vi "Create Control Addon.vi"(8 "error in (no error)":errorcluster, 11 "Name":string) -> (0 "error out":errorcluster, 3 "Custom Device Ref":refnum<k24>)   [LabVIEW 2013, in "Control SysDef API.lvlib"]
uses:
  Control SysDef API.lvlib
  NationalInstruments.VeriStand.SystemDefinitionAPI
  Shared/Constants.vi
  Shared/Control Addon Shared.lvlib
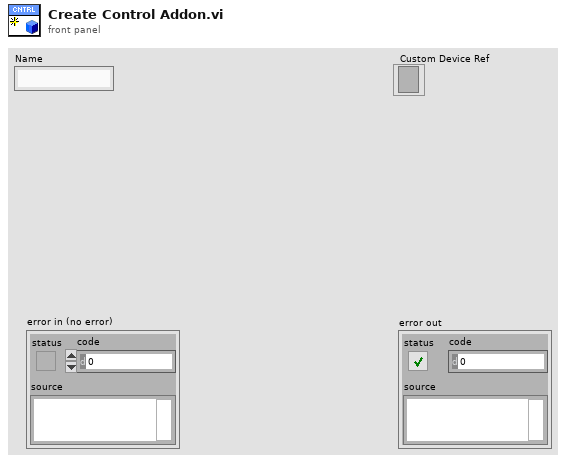
[diagram p1: front panel]
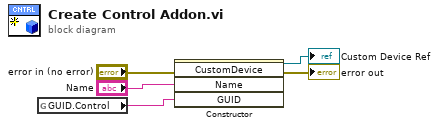
[diagram p0: block diagram]
diagram:
  n1 = global read "Constants.vi" "GUID.Control"() -> (w3:string)
  n2 = constructor class="CustomDevice"(error in="error in (no error)", "Name"="Name", "GUID"=w3) -> (reference out=→"Custom Device Ref":refnum<k24>, error out=→"error out":errorcluster)  [unwired: 2 in, 3 out]
